vi "Generate License File.vi"() -> ()   [LabVIEW 2015]
uses:
  Type/_Validation Period.ctl
panel:
  in  "Version Number (Optional)":string
  in  "Application Name":string="Simplicity 3Q Service"
  in  "Generate":bool
  in  "Valid For":T1=enum."3 Months"
  in  "Company / User Name":string="PerkinElmer"
  # "Please follow the following steps:  \n(1) enter a Company / User Name; \n(2) enter an optional Version Numver (if a version restriction is applied); \n(3) choose a desired Valid For period; \n(4) press the Generate File button;\n(5) copy the genated license file to the application folder."
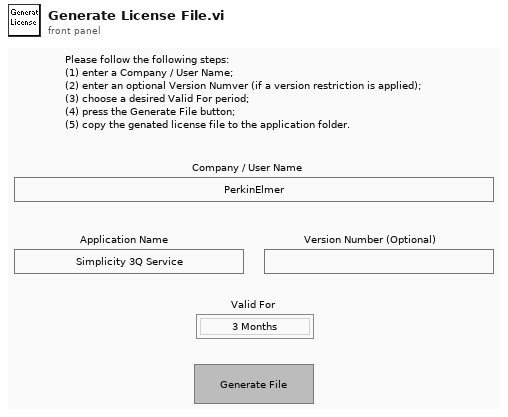
[diagram p1: front panel]
types:
  T1 = typedef "_Validation Period.ctl" = enum16{"1 Hour", "8 Hours", "1 Day", "1 Week", "1 Month", "3 Months", "6 Months", "1 year", "3 years", "Forever"}
  T2 = enum16{"open", "replace", "create", "open or create", "replace or create", "replace or create with confirmation"}
  T3 = cluster{"Company / User Name":string, "trimmed string":string, "Version Number (Optional)":string, dbl, dbl, "Key":string}
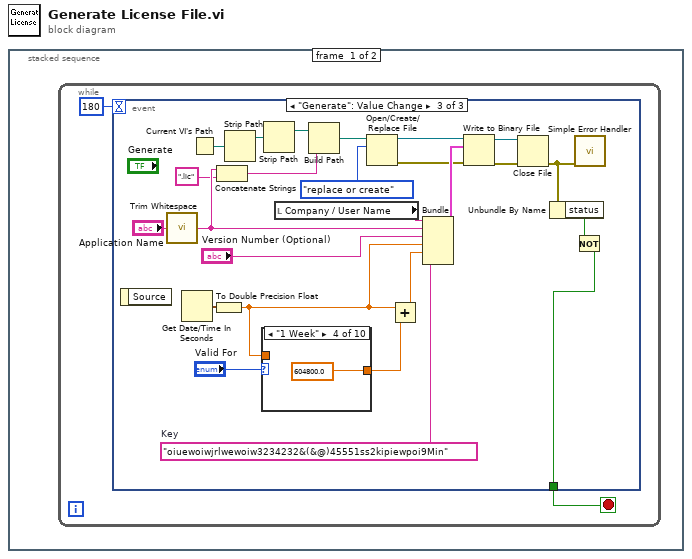
[diagram p0: block diagram]
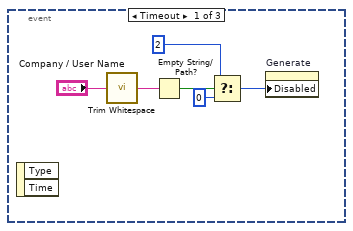
[diagram p2: hidden frame]
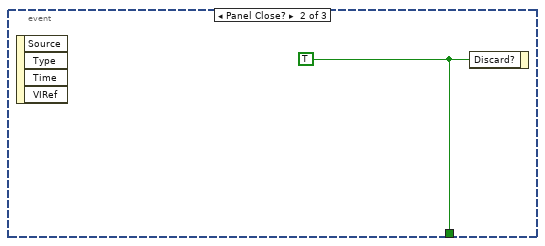
[diagram p3: hidden frame]
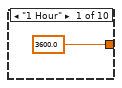
[diagram p4: hidden frame]
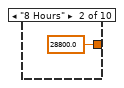
[diagram p5: hidden frame]
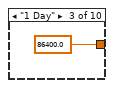
[diagram p6: hidden frame]
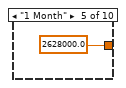
[diagram p7: hidden frame]
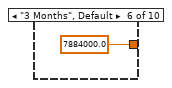
[diagram p8: hidden frame]
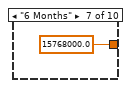
[diagram p9: hidden frame]
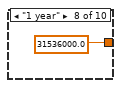
[diagram p10: hidden frame]
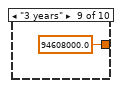
[diagram p11: hidden frame]
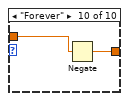
[diagram p12: hidden frame]
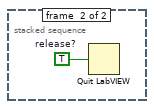
[diagram p13: hidden frame]
diagram:
  n1 = stacked-sequence {
    frame #0 {
      n2 = while {
        stop <- w1 stop-if-true
        n3 = event shown="[2] \"Generate\": Value Change" {
          selector: _ -> [_ _ _]
          dyn-events: _ -> [_ _ _]
          timeout: 180 -> [_ _ _]
          tunnel: [_ w9 w15] -> w1
          event Timeout {
            n4 = event-data() -> ()  [unwired: 3 out]
            n5 = call <vilib>:"Trim Whitespace.vi"("string"="Company / User Name") -> ("trimmed string"=w7:string)  [unwired: 1 in]
            n6 = Empty String/Path?(string/path=w7) -> (empty?=w6:bool)
            n7 = Select(t=u8 2 ("Disabled"), s=w6, f=u8 0) -> (s? t:f=w3:u8)
            n8 = property on="Generate" class="Bool"("Disabled"=w3) -> ()  [unwired: 2 in, 2 out]
          }
          event Panel Close? {
            w9 = TRUE ("Discard?")
            n9 = event-data() -> ()  [unwired: 5 out]
            n10 = event-data("Discard?"=w9) -> ()  [unwired: 1 in, 1 out]
          }
          event "Generate": Value Change {
            w14 = "oiuewoiwjrlwewoiw3234232&(&@)45551ss2kipiewpoi9Min"  # Key
            n11 = event-data() -> ()  [unwired: 2 out]
            n12 = call <vilib>:"Trim Whitespace.vi"("string"="Application Name") -> ("trimmed string"=w12:string)  [unwired: 1 in]
            n13 = Get Date/Time In Seconds() -> (seconds since 1Jan1904=w34:timestamp)
            n14 = Current VI's Path() -> (path=w26:path)
            n15 = To Double Precision Float(number=w34) -> (double precision float=w28:dbl)
            n16 = Concatenate Strings(w12, ".lic") -> (w10:string)
            n17 = Strip Path(path=w26) -> (stripped path=w27:path)  [unwired: 1 out]
            n18 = case shown="\"1 Week\"" "Valid For" {
              tunnel: [3600.0 28800.0 86400.0 604800.0 2628000.0 7884000.0 15768000.0 31536000.0 94608000.0 w45] -> w30
              tunnel: w28 -> [_ _ _ _ _ _ _ _ _ w44]
              frame "1 Hour" {
              }
              frame "8 Hours" {
              }
              frame "1 Day" {
              }
              frame "1 Week" {
              }
              frame "1 Month" {
              }
              frame "3 Months", Default {
              }
              frame "6 Months" {
              }
              frame "1 year" {
              }
              frame "3 years" {
              }
              frame "Forever" {
                n19 = Negate(x=w44) -> (-x=w45:dbl)
              }
            }
            n20 = Strip Path(path=w27) -> (stripped path=w25:path)  [unwired: 1 out]
            n21 = local read "Company / User Name"() -> (w31:string)
            n22 = Build Path(base path=w25, name or relative path=w10) -> (appended path=w24:path)
            n23 = Open/Create/Replace File(file path (use dialog)=w24, operation (0:open)=T2."replace or create") -> (refnum out=w22:refnum<file>, error out=w20:errorcluster)  [unwired: 1 in, 4 out]
            n24 = Add(x=w28, y=w30) -> (x+y=w29:dbl)
            n25 = Bundle("Company / User Name"=w31, "trimmed string"=w12, "Version Number (Optional)"="Version Number (Optional)", w28, w29, "Key"=w14) -> (w21:T3)  [unwired: 1 out]
            n26 = Write to Binary File(file (use dialog)=w22, data=w21, error in=w20) -> (refnum out=w18:refnum<file>, error out=w19:errorcluster)  [unwired: 4 out]
            n27 = Close File(refnum=w18, error in=w19) -> (error out=w17:errorcluster)  [unwired: 1 out]
            n28 = Unbundle By Name(w17) -> ("status"=w16:bool)
            n29 = Not(x=w16) -> (.not. x?=w15:bool)
            n30 = call <vilib>:"Simple Error Handler.vi"("error in (no error)"=w17) -> ()  [unwired: 1 in, 8 out]
          }
        }
      }
    }
    frame #1 {
      w46 = TRUE  # release?
      n31 = Quit LabVIEW(quit? (T)=w46) -> ()
    }
  }
